vi "niRFUtil TRC Trace to 2D DBL Array.vi"(7 "Measurement Trace":T1 format="%.2f") -> (8 "2D Array":sgl[][](array[numeric]) format="%.2f")   [LabVIEW 2015, in "niRFUtil.lvlib"]
uses:
  niRFUtil.lvlib
  Includes/niRFUtil INC Trace.ctl
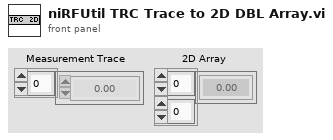
[diagram p1: front panel]
types:
  T1 = typedef "niRFUtil.lvlib/niRFUtil INC Trace.ctl" = sgl[]
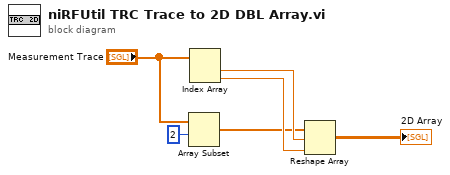
[diagram p0: block diagram]
diagram:
  n1 = Array Subset(array="Measurement Trace", index=2) -> (w3:T1)  [unwired: 1 in]
  n2 = Index Array(array="Measurement Trace") -> (element #1=w4:sgl, element #2=w5:sgl)  [unwired: 2 in]
  n3 = Reshape Array(w3, w4, w5) -> (→"2D Array":sgl[][])
